vi "hibakezelés.vi"(8 "error in (no error)":errorcluster, 11 "Enum in":T1) -> (0 "error out (no error)":errorcluster, 3 "Enum out":T1)   [LabVIEW 2016]
doc: "Hibakezelés."
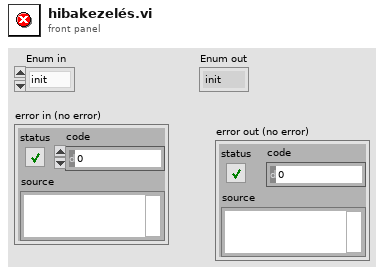
[diagram p1: front panel]
types:
  T1 = typedef "állapotok.ctl" = enum16{"init", "idle", "data load, filter, analysis", "filter", "analysis", "save", "save parameters", "load parameters", "stop"}
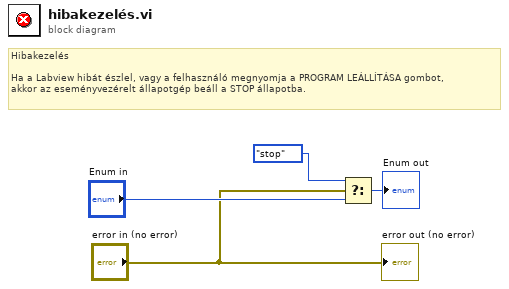
[diagram p0: block diagram]
diagram:
  # "Hibakezelés\n\nHa a Labview hibát észlel, vagy a felhasználó megnyomja a PROGRAM LEÁLLÍTÁSA gombot, \nakkor az eseményvezérelt állapotgép beáll a STOP állapotba."
  n1 = Select(t=állapotok."stop", s="error in (no error)", f="Enum in") -> (s? t:f=→"Enum out":T1)
  "error out (no error)" <- "error in (no error)"
